vi "Simple Semaphore.vi"() -> ()   [LabVIEW 2023]
doc: "This VI creates a semaphore and calls two parallel loops that will use the semaphore to update front panel data one at a time. Semaphores are most useful when you have parallel processes that need to access and \"lock\" a shared resource."
panel:
  out "Loop 2 Access?":bool
  out "Loop 1 Access?":bool
  out "Data 2":dbl(graph)
  out "Data 1":dbl(graph)
  in  "Stop":bool
  # "Overview: Demonstrates the use of the Semaphore VIs to control the execution of parallel code.\nInstructions:\nRun the VI."
  # "The Data chart will update for whichever loop has access. After a loop has access for 1 second, it will release the semaphore so the other loop can have access."
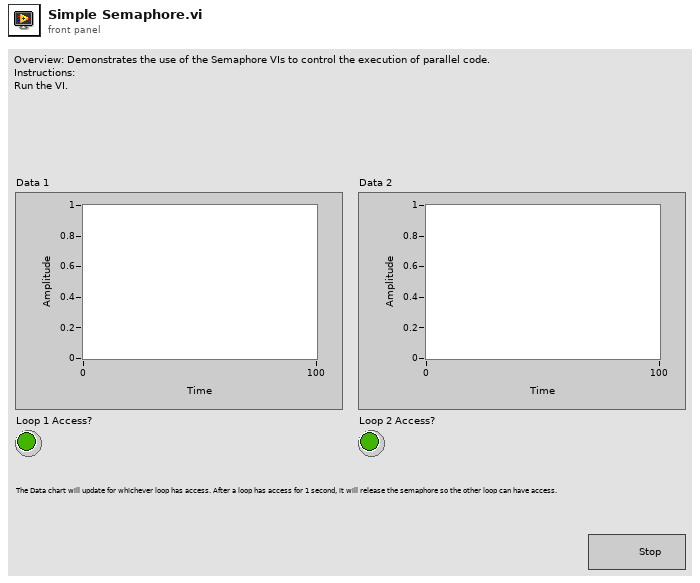
[diagram p1: front panel]
types:
  T1 = typedef "Semaphore RefNum" = refnum<k1>
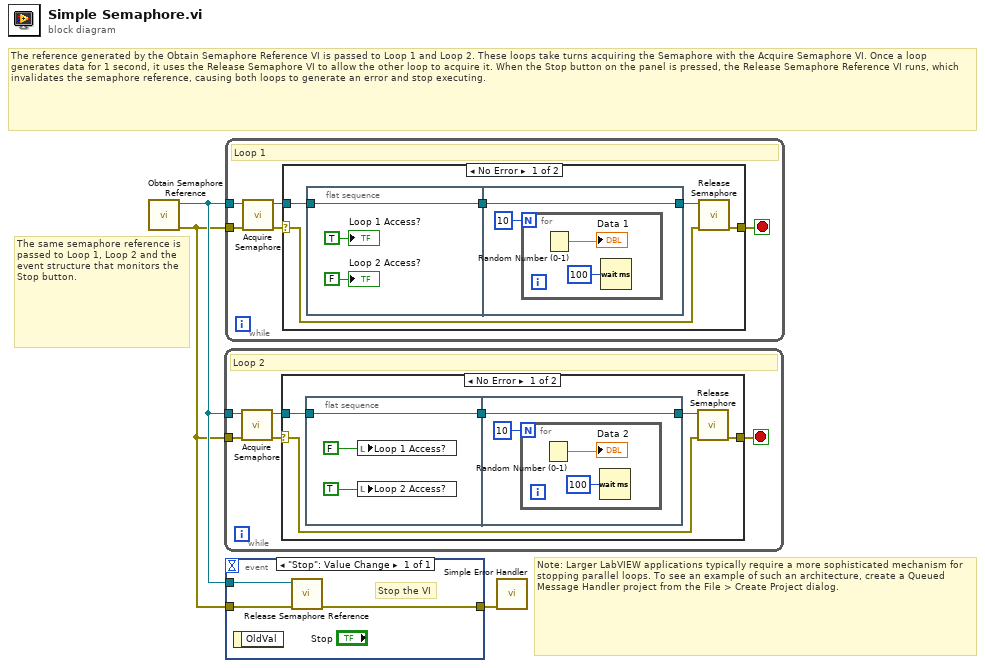
[diagram p0: block diagram]
diagram:
  # "Note: Larger LabVIEW applications typically require a more sophisticated mechanism for stopping parallel loops. To see an example of such an architecture, create a Queued Message Handler project from the File > Create Project dialog."
  # "The same semaphore reference is passed to Loop 1, Loop 2 and the event structure that monitors the Stop button."
  # "The reference generated by the Obtain Semaphore Reference VI is passed to Loop 1 and Loop 2. These loops take turns acquiring the Semaphore with the Acquire Semaphore VI. Once a loop generates data for 1 second, it uses the Release Semaphore VI to allow the other loop to acquire it. When the Stop button on the panel is pressed, the Release Semaphore Reference VI runs, which invalidates the semaphore reference, causing both loops to generate an error and stop executing."
  n1 = call <vilib>:"Obtain Semaphore Reference.vi"() -> ("error out"=w1:errorcluster, "semaphore"=w2:T1)  [unwired: 5 in, 1 out]
  n2 = while {
    tunnel: w2 -> [w8]
    tunnel: w1 -> [w7]
    stop <- w5 stop-if-true
    # "Loop 2"
    n3 = call <vilib>:"Acquire Semaphore.vi"("error in (no error)"=w7, "semaphore"=w8) -> ("error out"=w4:errorcluster, "semaphore out"=w6:T1)  [unwired: 3 in, 1 out]
    n4 = case shown="No Error" w4 {
      selector: w4 -> [w9 w21]
      tunnel: w6 -> [w12 _]
      tunnel: [w10 w21] -> w5
      frame No Error {
        n5 = flat-sequence {
          tunnel: w12 -> [w16]
          tunnel: [w16] -> w13
          tunnel: [w17] -> w11
          tunnel: w13 -> [w17]
          frame #0 {
            n6 = local write "Loop 1 Access?"(FALSE ("Loop 1 Access?")) -> ()
            n7 = local write "Loop 2 Access?"(TRUE ("Loop 2 Access?")) -> ()
          }
          frame #1 {
            n8 = for {
              N: 10 -> [_]
              n9 = Random Number (0-1)() -> (number: 0 to 1=→"Data 2":dbl)
              n10 = Wait (ms)(milliseconds to wait=u32 100) -> ()  [unwired: 1 out]
            }
          }
        }
        n11 = call <vilib>:"Release Semaphore.vi"("error in (no error)"=w9, "semaphore"=w11) -> ("error out"=w10:errorcluster)  [unwired: 4 in, 1 out]
      }
      frame Error {
        # "Semaphore reference was closed. Stop loop."
      }
    }
  }
  n12 = while {
    tunnel: w2 -> [w26]
    tunnel: w1 -> [w25]
    stop <- w23 stop-if-true
    # "Loop 1"
    n13 = call <vilib>:"Acquire Semaphore.vi"("error in (no error)"=w25, "semaphore"=w26) -> ("error out"=w22:errorcluster, "semaphore out"=w24:T1)  [unwired: 3 in, 1 out]
    n14 = case shown="No Error" w22 {
      selector: w22 -> [w27 w39]
      tunnel: w24 -> [w30 _]
      tunnel: [w28 w39] -> w23
      frame No Error {
        n15 = flat-sequence {
          tunnel: w30 -> [w32]
          tunnel: [w32] -> w31
          tunnel: [w35] -> w29
          tunnel: w31 -> [w35]
          frame #0 {
            "Loop 1 Access?" <- TRUE ("Loop 1 Access?")
            "Loop 2 Access?" <- FALSE ("Loop 2 Access?")
          }
          frame #1 {
            n16 = for {
              N: 10 -> [_]
              n17 = Random Number (0-1)() -> (number: 0 to 1=→"Data 1":dbl)
              n18 = Wait (ms)(milliseconds to wait=u32 100) -> ()  [unwired: 1 out]
            }
          }
        }
        n19 = call <vilib>:"Release Semaphore.vi"("error in (no error)"=w27, "semaphore"=w29) -> ("error out"=w28:errorcluster)  [unwired: 4 in, 1 out]
      }
      frame Error {
        # "Semaphore reference was closed. Stop loop."
      }
    }
  }
  n20 = event shown="[0] \"Stop\": Value Change" {
    selector: _ -> [_]
    dyn-events: _ -> [_]
    timeout: _ -> [_]
    tunnel: w1 -> [w41]
    tunnel: w2 -> [w42]
    tunnel: [w40] -> w3
    event "Stop": Value Change {
      # "Stop the VI"
      n21 = event-data() -> ()  [unwired: 1 in, 1 out]
      n22 = call <vilib>:"Release Semaphore Reference.vi"("error in (no error)"=w41, "semaphore"=w42) -> ("error out"=w40:errorcluster)  [unwired: 8 in, 1 out]
    }
  }
  n23 = call <vilib>:"Simple Error Handler.vi"("error in (no error)"=w3) -> ()  [unwired: 4 in, 5 out]
